vi "PID Voltage Sweep.vi"(8 "error in":errorcluster, 11 "classes in":T1) -> (0 "error out":errorcluster, 3 "classes out":T1)   [LabVIEW 2011]
uses:
  Controls/Class Objects.ctl
  Modules/File/Configuration/Configuration.lvclass
  Modules/Hardware/Power Supply/Power Supply.lvclass
  Modules/Hardware/Mass Flow Controller/Mass Flow Controller.lvclass
  Modules/Hardware/PID/PID.lvclass
  Modules/Hardware/Valve Controller/Valve Controller.lvclass
  Modules/Hardware/Multimeter/Multimeter.lvclass
  Modules/Hardware/Vapour Generator/Vapour Generator.lvclass
  Modules/File/TDMS/TDMS.lvclass
  Controls/User Interface Action.ctl
  Functional Global Data/Run Data.ctl
  Modules/Hardware/Mass Flow Controller/Flow Rate Units.ctl
  Functional Global Data/Device Params Global.ctl
  Functional Global Data/Globals.ctl
  Controls/TDMS File Handling.ctl
  Modules/Hardware/Power Supply/Source Units.ctl
  <vilib>/Platform/TimedLoop/XDataNode/timing_clust.ctl
  <vilib>/Platform/TimedLoop/XDataNode/nitl_modes.ctl
  <vilib>/Platform/TimedLoop/XDataNode/wakeup.ctl
  Modules/File/TDMS/File Level.ctl
  <vilib>/Platform/TimedLoop/XDataNode/XDataNode.xnode
  <vilib>/Platform/TimedLoop/XDataNode/XDNodeRunTimeDep.lvlib
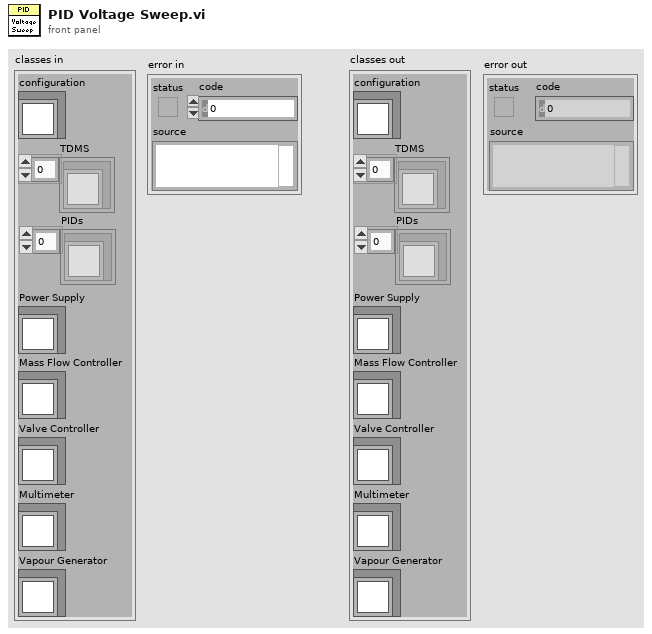
[diagram p1: front panel]
types:
  T1 = typedef "Class Objects.ctl" = cluster{"configuration":refnum<class "Configuration.lvclass">, "TDMS":refnum<class "TDMS.lvclass">[], "Power Supply":refnum<class "Power Supply.lvclass">, "Mass Flow Controller":refnum<class "Mass Flow Controller.lvclass">, "Valve Controller":refnum<class "Valve Controller.lvclass">, "Multimeter":refnum<class "Multimeter.lvclass">, "Vapour Generator":refnum<class "Vapour Generator.lvclass">, "PIDs":refnum<class "PID.lvclass">[]}
  T2 = typedef "User Interface Action.ctl" = enum16{"Initialize", "Data Acquisition Disable", "Data View Disable", "Sample Set", "Sample Set 2D Data", "Sample Set x0 & dx", "Sample Add", "Sample Set Cursor", "Sample Set Offset & Multiplier", "Sample Set Axis Labels", "Sample Parameters Disabled", "Sample Parameters Update", "Run Update", "Run Set Offset & Multiplier", "Run Set Axis Labels", "Run Set Cursor", "Run Set Disabled", "Run Parameters Update", "Run Parameters Disabled", "Run Number Set", "Run Number Set Range", "Run Number Set Disabled", "Sample Number Set", "Sample Number Set Range", "Notes Set Value", "Update Plot", "Set Plot Parameters", "Update Concentration Plot", "Time Set", "Clear DAQ Display", "Clear Analysis Display", "Status Bar Set", "Progress Bar Set", "Display Mode Set", "Experiment Type Set", "Analysis Plot Average Set", "Stop"}
  T3 = typedef "Device Params Global.ctl" = enum16{"Initialize", "Get Device Settings", "Get Device Connections", "Set Device Settings", "Set Device Connections", "Get All Device Properties"}
  T4 = typedef "Run Data.ctl" = enum16{"Initialize", "Add Sample Channel", "Set Run", "Get Number of Runs", "Set Run Params", "Get Spectrum", "Get Run Params", "Get Sample Params", "Get History", "Get Averaged History", "Get Run Param Names", "Set Run Param Names", "Get Sample Param Names", "Set Sample Param Names", "Get MFC Flow Rate Challenge Profile", "Get History Average"}
  T5 = typedef "Mass Flow Controller.lvclass/Flow Rate Units.ctl" = enum16{"ml/min"}
  T6 = typedef "Globals.ctl" = enum16{"Initialize", "Get DAQ Params", "Get Data Display Params", "Set DAQ Params", "Set Data Display Params"}
  T7 = typedef "TDMS File Handling.ctl" = enum16{"Add TDMS File", "Get Active TDMS File", "Set Active TDMS File", "Set Active TDMS File Index"}
  T8 = typedef "Power Supply.lvclass/Source Units.ctl" = enum16{"volts", "millivolts", "microvolts", "amps", "milliamps", "microamps", "nanoamps"}
  T9 = typedef "XDNodeRunTimeDep.lvlib/timing_clust.ctl" = cluster{"Expected End [f-1]":u64, "Actual End [f-1]":u64, "Finished Late? [f-1]":bool, "Expected End [i-1]":u64, "Actual End [i-1]":u64, "Finished Late? [i-1]":bool, "Expected Start [i]":u64, "Actual Start [i]":u64, "Expected Start [f]":u64, "Actual Start [f]":u64, "Source Name":string, "Structure Name":string, "Period":i64, "Deadline":i64, "Offset":i64, "Start":i64, "Priority":i32, "Timeout":i32, "Mode":T10, "Wakeup Reason":T11, "Error":errorcluster, "Source Type":string, "Secondary Source Type":string, "Global End Time":u64, "Global Start Time":u64, "Frame Duration":u64, "Iteration Duration":u64, "Assigned CPU":i32, "I/O Scan Engine Mode":u32}
  T10 = typedef "XDNodeRunTimeDep.lvlib/nitl_modes.ctl" = enum32{"No Change", "Process missed periods, maintain original phase", "Discard missed periods, maintain original phase", "Process missed periods, ignore original phase", "Discard missed periods, ignore original phase"}
  T11 = typedef "XDNodeRunTimeDep.lvlib/wakeup.ctl" = enum32{"Normal", "Aborted", "Asynchronous wakeup", "Timing source error", "Timed loop error", "Timeout"}
  T12 = typedef "TDMS.lvclass/File Level.ctl" = enum16{"File", "Group", "Channel"}
  T13 = typedef "Device Settings.ctl" = cluster{"PID":cluster{"B-M PID":T14, "INL PID":T15}, "Power Supply":cluster{"Source Value":dbl, "Source Value Units":T8, "Source Mode":T16, "Limits":T17, "Output":bool}, "Mass Flow Controller":cluster{"MFC Flow Rate":dbl, "MFC Valve Status":T20}, "Valve Controller":cluster{"Valve Assembly":T21}, "Multimeter":cluster{"Agilent 3458A":cluster{"Measurement Configuration":T23, "Measurement Integration":T24}}, "Vapour Generator":cluster{"Owlstone Permeation Tube":T25, "Owlstone GEN-SYS Setpoints":T27}}
  T14 = typedef "Baseline Mocon piD-Tech plus.lvclass/Settings.ctl" = cluster{"Detector Sampling Frequency":dbl}
  T15 = typedef "INL PID.lvclass/Settings.ctl" = cluster{"Sampling Frequency":dbl, "Integration Time":dbl, "Integration Periods":u8, "Grid Voltage":dbl}
  T16 = typedef "Power Supply.lvclass/Source Mode.ctl" = enum16{"Volts", "Current"}
  T17 = typedef "Power Supply.lvclass/Protection Limits.ctl" = cluster{"Voltage Limit":dbl, "Voltage Limit Units":T18, "Current Limit":dbl, "Current Limit Units":T19, "Voltage Trip/Cmpl":dbl, "Voltage Trip/Cmpl Units":T18, "Current Trip/Cmpl":dbl, "Current Trip/Cmpl Units":T19}
  T18 = typedef "Power Supply.lvclass/Voltage Units.ctl" = enum16{"volts", "millivolts", "microvolts"}
  T19 = typedef "Power Supply.lvclass/Current Units.ctl" = enum16{"amps", "milliamps", "microamps", "nanoamps"}
  T20 = typedef "Mass Flow Controller.lvclass/Valve Status.ctl" = enum16{"Open", "Closed"}
  T21 = typedef "Valve Controller.lvclass/Valve Assembly.ctl" = cluster{"Valve 1":T22, "Valve 2":T22, "Valve 3":T22, "Valve 4":T22, "Valve 5":T22}
  T22 = typedef "Valve Controller.lvclass/Status.ctl" = u16
  T23 = typedef "Agilent 3458A.lvclass/Measurement Configuration.ctl" = cluster{"Function":enum16{"DC Voltage", "AC Voltage", "AC + DC Voltage", "DC Current", "AC Current", "AC + DC Current", "2-Wire Resistance", "4-Wire Resistance", "Frequency", "Period", "Direct Sampling DC", "Direct Sampling AC", "Sub-Sampling DC", "Sub-Sampling AC"}, " Manual Resolution":enum16{"4.5", "5.5", "6.5", "7.5", "8.5"}, "Frequency Source":enum16{"AC + DC Current", "AC + DC Voltage", "AC Current", "AC Voltage"}, "Auto Range":enum16{"OFF", "ON", "ONCE"}}
  T24 = typedef "Agilent 3458A.lvclass/Measurement Integration.ctl" = cluster{"Power Line Cycles":dbl}
  T25 = typedef "Owlstone GEN-SYS.lvclass/Permeation Tube.ctl" = cluster{"Tube":T26, "Molecular Weight":dbl, "Calibration Temperature\n(Celcius)":i32, "Permeation Rate \n(ng/min)":i32}
  T26 = typedef "Owlstone GEN-SYS.lvclass/Permeation Tube Gas.ctl" = enum16{"Isobutylene 27 Nov 2012", "Ammonia 29 Sep 2012", "DMMP Tube A 3 July 2014", "DMMP Tube B 3 July 2014"}
  T27 = typedef "Owlstone GEN-SYS.lvclass/Gen-Sys Setpoints.ctl" = cluster{"OVG-4":cluster{"Oven Temperature":i32, "Sample Flow Rate":i32, "Split Flow Status":u16, "Split Flow Rate":i32}, "OHG-4":cluster{"Wet Air Flow":i32}}
  T28 = typedef "Data Acquisition Parameters.ctl" = cluster{"Experiment Type":T29, "Experiment Name":string, "Operator Name":string, "Notes":string, "TDMS File Path":path, "Data Acquisition State":bool, "PID Voltage Sweep":T30, "MFC Challenge Profile - Heaviside Step":T31, "MFC Challenge Profile":T32, "MFC Challenge Profile - Staircase":T33}
  T29 = typedef "DAQ Type.ctl" = enum16{"PID Sample", "PID with PS Challenge", "PID with MFC Challenge", "Multimeter Sample", "Multimeter with MFC Challenge"}
  T30 = typedef "PID Voltage Seep Settings.ctl" = cluster{"Voltage Step (V)":dbl, "Voltage Range (V)":cluster{u16, u16}, "Time Step (s)":dbl, "Voltage Step Direction":enum16{"High 2 Low", "Low 2 High"}}
  T31 = typedef "MFC Challenge Profile - Heaviside Step.ctl" = cluster{"Valve Open Duration":u16, "MFC Flow Rate":dbl, "Valve Open Repeats":u16, "Valve Open Start":u16}
  T32 = typedef "MFC Challen Profile Type.ctl" = enum16{"Heaviside", "Staircase"}
  T33 = typedef "MFC Challenge Profile - Staircase.ctl" = cluster{"Step Time Duration":u16, "Step Flow Rate":dbl, "Steps":u16, "Valve Open Start":u16, "Recovery":bool, "Repeats":u16}
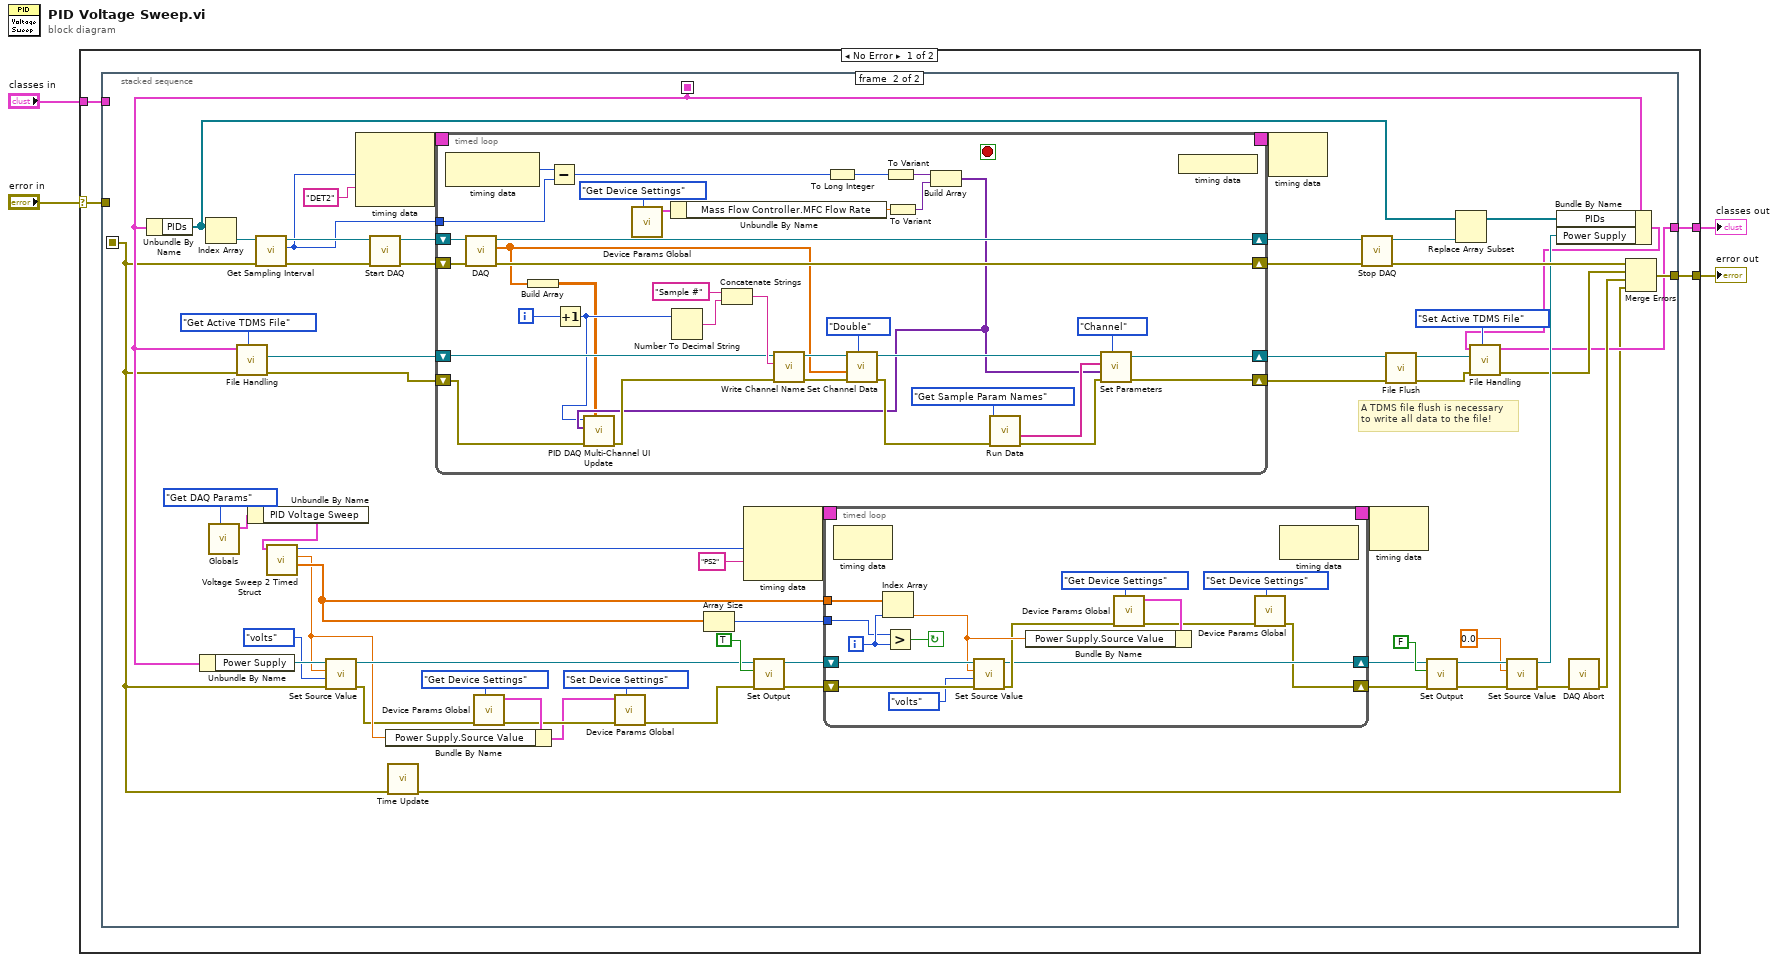
[diagram p0: block diagram]
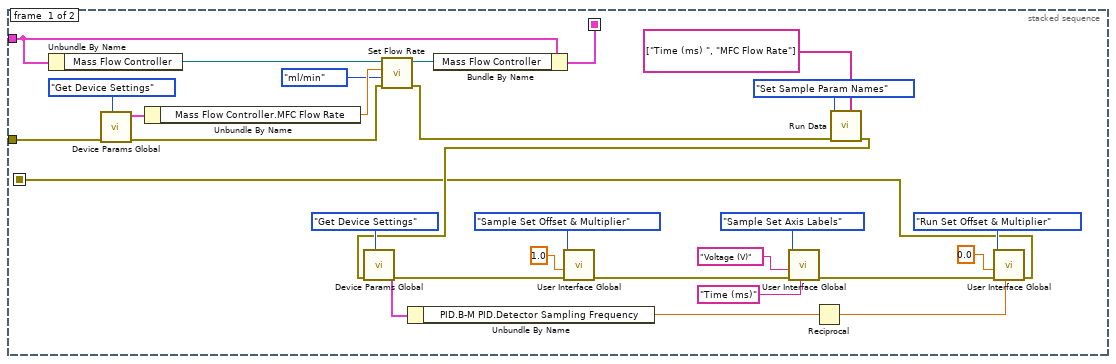
[diagram p2: hidden frame]
diagram:
  n1 = case shown="No Error" "error in" {
    selector: "error in" -> [w5 w166]
    tunnel: [w8 w166] -> w4
    tunnel: "classes in" -> [w7 w165]
    tunnel: [w6 w165] -> w1
    frame No Error {
      n2 = stacked-sequence {
        seq-local: [w10 _] -> [_ w44]
        seq-local: [w28 _] -> [_ w54]
        tunnel: [_ w84] -> w8
        tunnel: w7 -> [w30 _]
        tunnel: [_ w48] -> w6
        tunnel: w5 -> [w36 _]
        frame #0 {
          n3 = Unbundle By Name(w30) -> ("Mass Flow Controller"=w34:refnum<class "Mass Flow Controller.lvclass">)
          n4 = call "Device Params Global.vi"("action"=Device_Params_Global."Get Device Settings", "error in"=w36) -> ("error out"=w32:errorcluster, "Device Settings OUT"=w35:T13)  [unwired: 7 in, 1 out]
          n5 = Unbundle By Name(w35) -> ("Mass Flow Controller.MFC Flow Rate"=w33:dbl)
          n6 = call-dynamic "Set Flow Rate.vi"("error in (no error)"=w32, "Flow Rate Units"=Flow_Rate_Units."ml/min", "Flow Rate"=w33, "Mass Flow Controller in"=w34) -> ("error out"=w25:errorcluster, "Mass Flow Controller out"=w29:refnum<class "Mass Flow Controller.lvclass">)  [unwired: 6 in]
          n7 = Bundle By Name(cluster=w30, "Mass Flow Controller"=w29) -> (w28:T1)
          n8 = call "Run Data.vi"("Param Names IN"=string[] ["Time (ms) ", "MFC Flow Rate"] ("Sample Parm Names"), "error in"=w25, "action"=Run_Data."Set Sample Param Names") -> ("error out"=w11:errorcluster)  [unwired: 5 in, 3 out]
          n9 = call "Device Params Global.vi"("action"=Device_Params_Global."Get Device Settings", "error in"=w11) -> ("error out"=w24:errorcluster, "Device Settings OUT"=w23:T13)  [unwired: 7 in, 1 out]
          n10 = Unbundle By Name(w23) -> ("PID.B-M PID.Detector Sampling Frequency"=w14:dbl)
          n11 = call "User Interface Global.vi"("error in"=w24, "data1"=1.0, "action"=User_Interface_Action."Sample Set Offset & Multiplier" ("Action")) -> ("error out"=w18:errorcluster)  [unwired: 8 in]
          n12 = call "User Interface Global.vi"("data2"="Time (ms)", "error in"=w18, "data1"="Voltage (V)", "action"=User_Interface_Action."Sample Set Axis Labels" ("Action")) -> ("error out"=w13:errorcluster)  [unwired: 7 in]
          n13 = Reciprocal(x=w14) -> (1/x=w9:dbl)
          n14 = call "User Interface Global.vi"("data2"=w9, "error in"=w13, "data1"=0.0 ("1/x"), "action"=User_Interface_Action."Run Set Offset & Multiplier" ("Action")) -> ("error out"=w10:errorcluster)  [unwired: 7 in]
        }
        frame #1 {
          # "A TDMS file flush is necessary\nto write all data to the file!"
          n15 = Unbundle By Name(w54) -> ("PIDs"=w40:refnum<class "PID.lvclass">[])
          n16 = Unbundle By Name(w54) -> ("Power Supply"=w67:refnum<class "Power Supply.lvclass">)
          n17 = Index Array(array=w40) -> (element=w41:refnum<class "PID.lvclass">)  [unwired: 1 in]
          n18 = call "Globals.vi"("action"=Globals."Get DAQ Params") -> ("Data Acquisition"=w46:T28)  [unwired: 8 in, 2 out]
          n19 = call "File Handling.vi"("TDMS File Handling"=TDMS_File_Handling."Get Active TDMS File", "error in"=w44, "Class objects"=w54) -> ("error out"=w90:errorcluster, "TDMS File"=w93:refnum<class "TDMS.lvclass">)  [unwired: 6 in, 1 out]
          n20 = Unbundle By Name(w46) -> ("PID Voltage Sweep"=w45:T30)
          n21 = call-dynamic "Get Sampling Interval.vi"("error in (no error)"=w44, "PID in"=w41) -> ("error out"=w83:errorcluster, "Sampling Interval"=w42:u32, "PID out"=w82:refnum<class "PID.lvclass">)  [unwired: 7 in]
          n22 = call "Voltage Sweep 2 Timed Struct.vi"("Voltage Sweep Settings"=w45) -> ("Vector"=w74:dbl[], "V0"=w62:dbl, "dT"=w75:i32)  [unwired: 8 in]
          n23 = call-dynamic "Set Source Value.vi"("error in (no error)"=w44, "Source Value Units"=Source_Units."volts", "Source Value"=w62, "Power Supply in"=w67) -> ("error out"=w61:errorcluster, "Power Supply out"=w72:refnum<class "Power Supply.lvclass">)  [unwired: 6 in]
          n24 = node-c288(w42, "DET2" ("Name")) -> (w99:T9)  [unwired: 1 in]
          n25 = call-dynamic "Start DAQ.vi"("error in (no error)"=w83, "Detector in"=w82) -> ("error out"=w88:errorcluster, "Detector out"=w89:refnum<class "PID.lvclass">)  [unwired: 8 in]
          n26 = call "Time Update.vi"("error in"=w44) -> ("error out"=w43:errorcluster)  [unwired: 10 in]
          n27 = timed-loop {
            timing: w99 -> [_]
            timing-out: [_] -> w98
            shift-right: [w154] -> w87
            shift-left: w89 -> [w156]
            shift-right: [w137] -> w91
            shift-left: w90 -> [w138]
            shift-right: [w136] -> w92
            shift-left: w93 -> [w139]
            shift-right: [w153] -> w86
            shift-left: w88 -> [w155]
            tunnel: w42 -> [w128]
            i -> [w124]
            stop <- _ stop-if-true
            n28 = node-c288() -> (w129:i64)  [unwired: 1 in]
            n29 = call-dynamic "DAQ.vi"("error in"=w155, "Detector in"=w156) -> ("error out"=w153:errorcluster, "data"=w123:dbl[], "Detector out"=w154:refnum<class "PID.lvclass">)  [unwired: 7 in]
            n30 = Build Array(w123) -> (w122:dbl[][])
            n31 = Subtract(x=w129, y=w128) -> (x-y=w127:i64)
            n32 = Increment(x=w124) -> (x+1=w125:i32)
            n33 = call "Device Params Global.vi"("action"=Device_Params_Global."Get Device Settings") -> ("Device Settings OUT"=w134:T13)  [unwired: 8 in, 2 out]
            n34 = Unbundle By Name(w134) -> ("Mass Flow Controller.MFC Flow Rate"=w133:dbl)
            n35 = Number To Decimal String(number=w125) -> (decimal integer string=w149:string)  [unwired: 1 in]
            n36 = Concatenate Strings("Sample #" ("string"), w149) -> (w147:string)
            n37 = To Long Integer(number=w127) -> (32bit integer=w130:i32)
            n38 = To Variant(anything=w130) -> (Variant=w131:variant)
            n39 = To Variant(anything=w133) -> (Variant=w132:variant)
            n40 = Build Array(w131, w132) -> (w126:variant[])
            n41 = call "PID DAQ Multi-Channel UI Update.vi"("Sample Data"=w122, "error in"=w138, "Sample Parameter"=w126, "Sample Number"=w125) -> ("error out"=w150:errorcluster)  [unwired: 7 in]
            n42 = call-dynamic "Write Channel Name.vi"("error in (no error)"=w150, "Channel Name"=w147, "TDMS in"=w139) -> ("error out"=w142:errorcluster, "TDMS out"=w145:refnum<class "TDMS.lvclass">)  [unwired: 7 in]
            n43 = call-dynamic "Set Channel Data.vi"("data type"=enum16{"I16", "Double"}."Double" ("Data Type"), "error in"=w142, "double channel data"=w123, "TDMS in"=w145) -> ("error out"=w151:errorcluster, "TDMS out"=w144:refnum<class "TDMS.lvclass">)  [unwired: 6 in]
            n44 = call "Run Data.vi"("error in"=w151, "action"=Run_Data."Get Sample Param Names" ("Action")) -> ("error out"=w152:errorcluster, "Param Names OUT"=w140:string[])  [unwired: 6 in, 2 out]
            n45 = call-dynamic "Set Parameters.vi"("File Level"=File_Level."Channel", "error in (no error)"=w152, "property values"=w126, "property names"=w140, "TDMS.lvclass in"=w144) -> ("error out"=w137:errorcluster, "TDMS.lvclass out"=w136:refnum<class "TDMS.lvclass">)  [unwired: 5 in]
            n46 = node-c288() -> ()  [unwired: 1 out]
          }
          n47 = call "Device Params Global.vi"("action"=Device_Params_Global."Get Device Settings", "error in"=w61) -> ("error out"=w59:errorcluster, "Device Settings OUT"=w63:T13)  [unwired: 7 in, 1 out]
          n48 = Bundle By Name(cluster=w63, "Power Supply.Source Value"=w62) -> (w58:T13)
          n49 = call "Device Params Global.vi"("action"=Device_Params_Global."Set Device Settings", "error in"=w59, "Device Settings IN"=w58) -> ("error out"=w57:errorcluster)  [unwired: 6 in, 2 out]
          n50 = Array Size(array=w74) -> (size(s)=w73:i32)
          n51 = node-c288(w75, "PS2" ("Structure Name")) -> (w97:T9)  [unwired: 1 in]
          n52 = call-dynamic "Set Output.vi"("error in (no error)"=w57, "Enable"=TRUE ("Status"), "Power Supply in"=w72) -> ("error out"=w78:errorcluster, "Power Supply out"=w79:refnum<class "Power Supply.lvclass">)  [unwired: 7 in]
          n53 = timed-loop {
            timing: w97 -> [_]
            timing-out: [_] -> w96
            tunnel: w74 -> [w112]
            tunnel: w73 -> [w111]
            shift-right: [w101] -> w56
            shift-left: w79 -> [w109]
            shift-right: [w100] -> w55
            shift-left: w78 -> [w110]
            i -> [w113]
            stop <- w114 continue-if-true
            n54 = node-c288() -> ()  [unwired: 1 in, 1 out]
            n55 = Index Array(array=w112, index=w113) -> (element=w103:dbl)
            n56 = Greater?(x=w111, y=w113) -> (0:w114:bool)
            n57 = call-dynamic "Set Source Value.vi"("error in (no error)"=w110, "Source Value Units"=Source_Units."volts", "Source Value"=w103, "Power Supply in"=w109) -> ("error out"=w102:errorcluster, "Power Supply out"=w101:refnum<class "Power Supply.lvclass">)  [unwired: 6 in]
            n58 = call "Device Params Global.vi"("action"=Device_Params_Global."Get Device Settings", "error in"=w102) -> ("error out"=w104:errorcluster, "Device Settings OUT"=w106:T13)  [unwired: 7 in, 1 out]
            n59 = Bundle By Name(cluster=w106, "Power Supply.Source Value"=w103) -> ()  [unwired: 1 out]
            n60 = call "Device Params Global.vi"("action"=Device_Params_Global."Set Device Settings", "error in"=w104) -> ("error out"=w100:errorcluster)  [unwired: 7 in, 2 out]
            n61 = node-c288() -> ()  [unwired: 1 in, 1 out]
          }
          n62 = node-c288(w98) -> ()  [unwired: 1 out]
          n63 = call-dynamic "Stop DAQ.vi"("error in (no error)"=w86, "Detector in"=w87) -> ("error out"=w85:errorcluster, "Detector out"=w39:refnum<class "PID.lvclass">)  [unwired: 8 in]
          n64 = node-c288(w96) -> ()  [unwired: 1 out]
          n65 = call-dynamic "File Flush.vi"("error in"=w91, "TDMS in"=w92) -> ("error out"=w51:errorcluster, "TDMS out"=w52:refnum<class "TDMS.lvclass">)  [unwired: 8 in]
          n66 = call-dynamic "Set Output.vi"("error in (no error)"=w55, "Enable"=FALSE ("Status"), "Power Supply in"=w56) -> ("error out"=w71:errorcluster, "Power Supply out"=w70:refnum<class "Power Supply.lvclass">)  [unwired: 7 in]
          n67 = Replace Array Subset(array=w40, new element=w39) -> (w38:refnum<class "PID.lvclass">[])  [unwired: 1 in]
          n68 = call-dynamic "Set Source Value.vi"("error in (no error)"=w71, "Source Value"=0.0 ("Voltage"), "Power Supply in"=w70) -> ("error out"=w68:errorcluster, "Power Supply out"=w69:refnum<class "Power Supply.lvclass">)  [unwired: 7 in]
          n69 = Bundle By Name(cluster=w54, "PIDs"=w38, "Power Supply"=w69) -> (w49:T1)
          n70 = call "File Handling.vi"("TDMS File Handling"=TDMS_File_Handling."Set Active TDMS File", "error in"=w51, "TDMS File"=w52, "Class objects"=w49) -> ("error out"=w50:errorcluster, "Class objects"=w48:T1)  [unwired: 5 in, 1 out]
          n71 = call "DAQ Abort.vi"("error in"=w68) -> ("error out"=w76:errorcluster)  [unwired: 9 in]
          n72 = Merge Errors(w85, w50, w76, w43) -> (w84:errorcluster)
        }
      }
    }
    frame Error {
    }
  }
  "error out" <- w4
  "classes out" <- w1
